vi "Check for Duplicate Variables.vi"(7 "Command/Response Refnum in":T1 format="%.0x", 8 "error in (no error)":errorcluster, 11 "Command/Response Format in":string) -> (0 "error out":errorcluster, 2 "Variables":string[](array[string]), 3 "Command/Response Format out":string)   [LabVIEW 2018, in "Instrument Addon Scripting API.lvlib"]
uses:
  Instrument Addon Scripting API.lvlib
  <vilib>/NI Veristand/Custom Device API/Custom Device Item Ref.ctl
  Addon/Addon Shared/SubVIs/Constants.vi
  Addon/Addon System Explorer/Instrument Addon System Explorer.lvlib
  Addon/Addon Shared/Instrument Addon Shared.lvlib
  <vilib>/NI VeriStand/Custom Device API/Custom Device API.lvlib
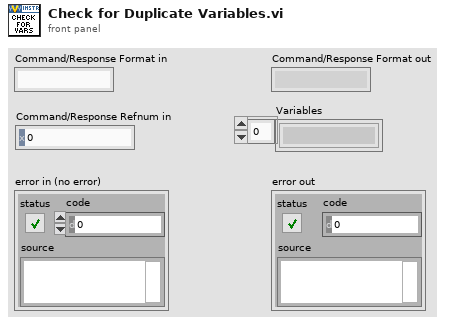
[diagram p1: front panel]
types:
  T1 = typedef "Custom Device API.lvlib/Custom Device Item Ref.ctl" = u64
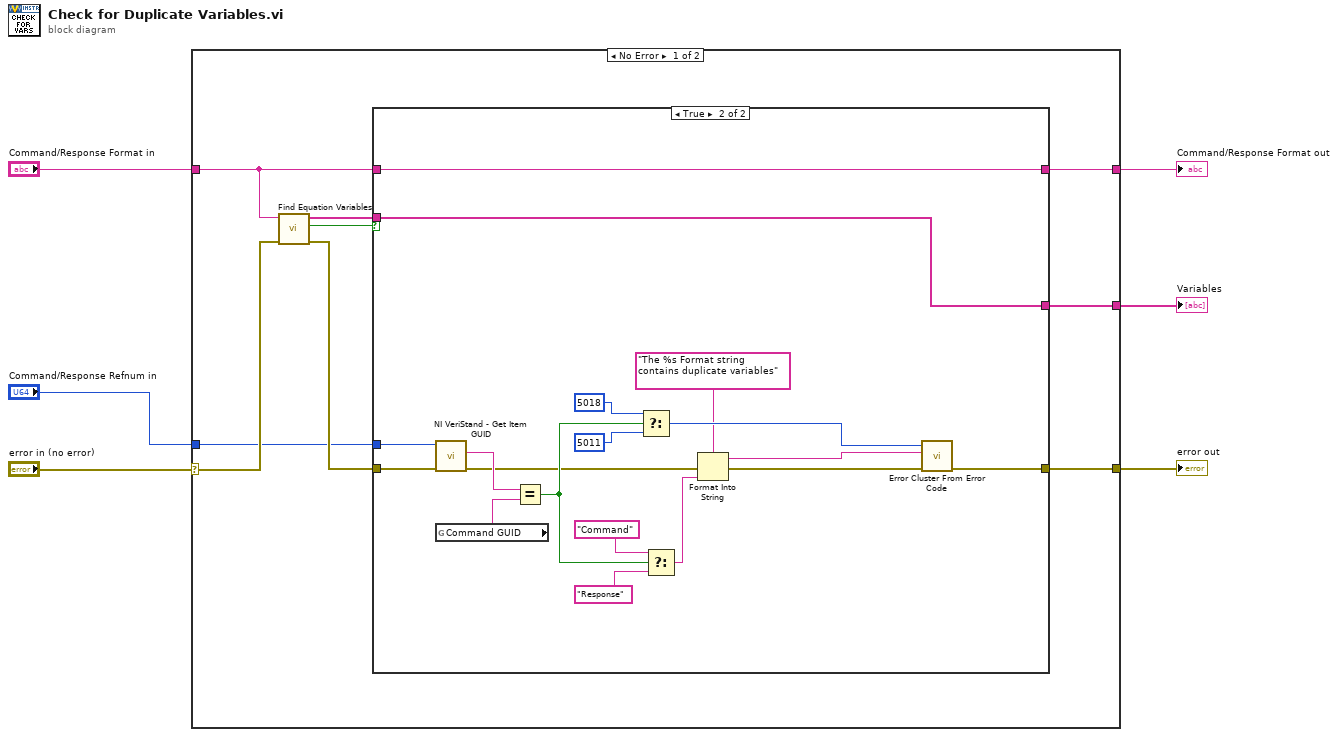
[diagram p0: block diagram]
diagram:
  n1 = case shown="No Error" "error in (no error)" {
    selector: "error in (no error)" -> [w8 w38]
    tunnel: [w13 w38] -> w6
    tunnel: [w11 _] -> w5
    tunnel: "Command/Response Format in" -> [w10 w37]
    tunnel: [w9 w37] -> w3
    tunnel: "Command/Response Refnum in" -> [w7 _]
    frame No Error {
      n2 = call "Find Equation Variables.vi"("error in (no error)"=w8, "Command"=w10) -> ("error out"=w14:errorcluster, "Duplicate?"=w15:bool, "Variables"=w12:string[])  [unwired: 7 in]
      n3 = case shown="True" w15 {
        tunnel: w14 -> [w18 w24]
        tunnel: [w18 w36] -> w13
        tunnel: w12 -> [w16 w35]
        tunnel: [w16 w35] -> w11
        tunnel: w10 -> [w17 w34]
        tunnel: [w17 w34] -> w9
        tunnel: w7 -> [_ w19]
        frame False {
        }
        frame True {
          n4 = call <vilib>:"NI VeriStand - Get Item GUID.vi"("error in (no error)"=w24, "Item Ref in"=w19) -> ("error out"=w30:errorcluster, "GUID"=w31:string)  [unwired: 7 in, 1 out]
          n5 = global read "Constants.vi" "Command GUID"() -> (w32:string)
          n6 = Equal?(x=w31, y=w32) -> (x = y?=w33:bool)
          n7 = Select(t=5018 ("error code (0)"), s=w33, f=5011 ("error code (0)")) -> (s? t:f=w22:i32)
          n8 = Select(t="Command", s=w33, f="Response") -> (s? t:f=w29:string)
          n9 = Format Into String(format string="The %s Format string contains duplicate variables" ("error message (\"\")"), error in=w30, w29) -> (resulting string=w21:string, error out=w23:errorcluster)  [unwired: 1 in]
          n10 = call <vilib>:"Error Cluster From Error Code.vi"("error in (no error)"=w23, "error message (\"\")"=w21, "error code (0)"=w22) -> ("error out"=w36:errorcluster)  [unwired: 6 in]
        }
      }
    }
    frame Error {
    }
  }
  "error out" <- w6
  "Variables" <- w5
  "Command/Response Format out" <- w3
